vi "Neutral_Agilent_E3631A_TriggerSet_v2_20151211.vi"(5 "Triggeed Current Limit":dbl[](array[numeric]) format="%.2g", 6 "Program Trigger?":bool[](array[boolean]), 7 "Triggerd Voltage Level":dbl[](array[numeric]) format="%.3g", 8 "error in (no error)":errorcluster={"status"=FALSE, "code"=0, "source"="gettemp.vi: No error - function call successful"}, 9 "Trigger Delay (s)":dbl min=0.0 max=3600.0 step=1.0 format="%.2f", 10 "Channel":i32[](array[ring]) items=["+6V"=1, "+24V"=2, "-24V"=3], 11 "VISA resource name":refnum<visa-resource-name>) -> (0 "error out":errorcluster={"status"=TRUE, "code"=-1074000000, "source"="Agilent E363X Series.lvlib:Error Query.vi<ERR>\nInstrument reports:\n-222,\"Data out of range\"\r\n+0,\"No error\"\r\n\n\n\n<b>Complete call chain:</b>\r\n     Agilent E363X Series.lvlib:Error Query.vi\r\n     Agilent E363X Series.lvlib:Configure Output.vi\r\n     Neutral_Agilent_E3631A_20151027.vi\r\n     RydbergExpControl.vi"})   [LabVIEW 2016]
doc: "This example demonstrates the triggering functionality of the power supply. Initial and triggered voltage and limit settings are configured. The Send Software Trigger VI is used to trigger the instrument."
uses:
  Agilent Driver/Agilent E363X Series.lvlib
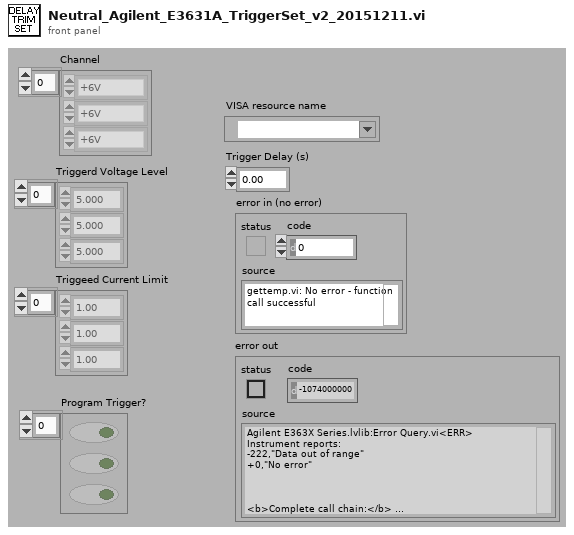
[diagram p1: front panel]
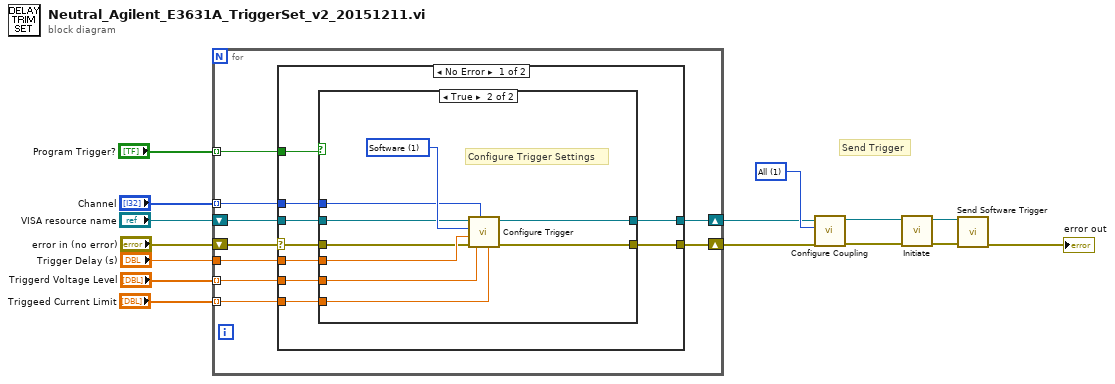
[diagram p0: block diagram]
diagram:
  w7 = u16 1 items=["None", "All", "Channels 1 & 2", "Channels 1 & 3", "Channels 2 & 3"] ("Coupling Setting (1: All)")
  # "Send Trigger"
  n1 = for {
    tunnel: "Triggerd Voltage Level" -> [w23] mode=indexing
    tunnel: "Triggeed Current Limit" -> [w22] mode=indexing
    tunnel: "Trigger Delay (s)" -> [w21]
    shift-right: [w24] -> w5
    shift-left: "error in (no error)" -> [w16]
    tunnel: "Channel" -> [w20] mode=indexing
    shift-right: [w18] -> w6
    shift-left: "VISA resource name" -> [w19]
    tunnel: "Program Trigger?" -> [w17] mode=indexing
    n2 = case shown="No Error" w16 {
      selector: w16 -> [w25 w46]
      tunnel: [w33 w46] -> w24
      tunnel: w23 -> [w32 _]
      tunnel: w22 -> [w31 _]
      tunnel: w21 -> [w30 _]
      tunnel: w20 -> [w29 _]
      tunnel: w19 -> [w28 w45]
      tunnel: [w27 w45] -> w18
      tunnel: w17 -> [w26 _]
      frame No Error {
        n3 = case shown="True" w26 {
          tunnel: [w34 w36] -> w33
          tunnel: w32 -> [_ w43]
          tunnel: w31 -> [_ w42]
          tunnel: w30 -> [_ w41]
          tunnel: w25 -> [w34 w40]
          tunnel: w29 -> [_ w39]
          tunnel: w28 -> [w35 w38]
          tunnel: [w35 w37] -> w27
          frame False {
          }
          frame True {
            w44 = u16 1 items=["Immediate", "Software"] ("Trigger Source (0: Immediate)")
            # "Configure Trigger Settings"
            n4 = call "Configure Trigger.vi"("Triggered Current Limit (0.0 A)"=w42, "Triggered Voltage Level (0.0 V)"=w43, "Channel (1: Channel 1)"=w39, "error in (no error)"=w40, "Trigger Delay (0 sec)"=w41, "Trigger Source (0: Immediate)"=w44, "VISA resource name"=w38) -> ("error out"=w36:errorcluster, "VISA resource name out"=w37:refnum<visa-resource-name>)  [unwired: 3 in]
          }
        }
      }
      frame Error {
      }
    }
  }
  n5 = call "Configure Coupling.vi"("error in (no error)"=w5, "Coupling Setting (1: All)"=w7, "VISA resource name"=w6) -> ("error out"=w3:errorcluster, "VISA resource name out"=w4:refnum<visa-resource-name>)  [unwired: 7 in]
  n6 = call "Initiate.vi"("error in (no error)"=w3, "VISA resource name"=w4) -> ("error out"=w1:errorcluster, "VISA resource name out"=w2:refnum<visa-resource-name>)  [unwired: 8 in]
  n7 = call "Send Software Trigger.vi"("error in (no error)"=w1, "VISA resource name"=w2) -> ("error out"=→"error out":errorcluster)  [unwired: 8 in, 1 out]
